vi "Destroy Events.vi"(8 "error in (no error)":errorcluster, 11 "RPI.SenseHat.Actor in":refnum<class "RPI.SenseHat.Actor.lvclass">) -> (0 "error out":errorcluster, 3 "RPI.SenseHat.Actor out":refnum<class "RPI.SenseHat.Actor.lvclass">)   [LabVIEW 2020, in "RPI.SenseHat.Actor.lvlib" / "RPI.SenseHat.Actor.lvclass"]
uses:
  RPI.SenseHat.Actor.lvclass
  RPI.SenseHat.Actor.lvclass/RPI.SenseHat.Actor.ctl
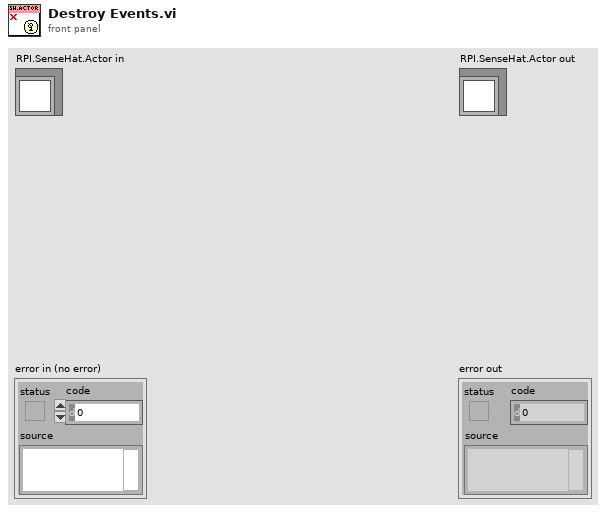
[diagram p1: front panel]
types:
  T1 = typedef "RPI.SenseHat.Actor.lvlib/RPI.SenseHat.Actor.lvclass/Public Events.ctl" = cluster{"Joystick Update":refnum<user-event>}
  T2 = typedef "RPI.SenseHat.Actor.lvlib/RPI.SenseHat.Actor.lvclass/Protected Events.ctl" = cluster{"StopActor":refnum<user-event>}
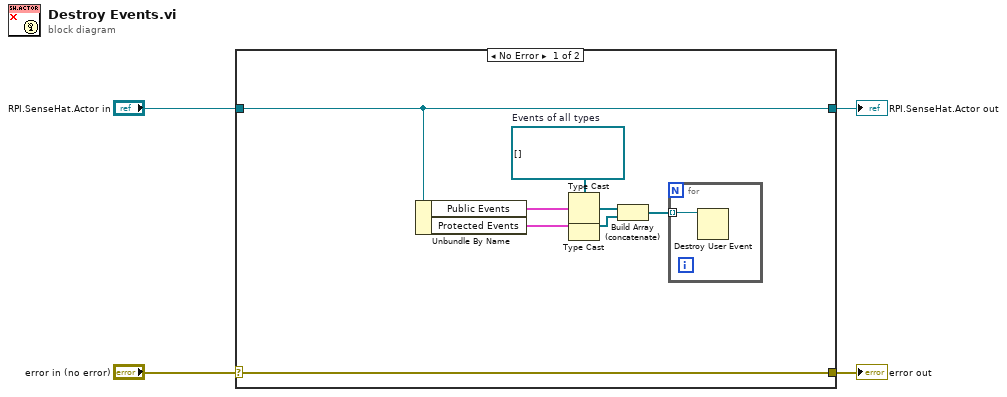
[diagram p0: block diagram]
diagram:
  n1 = case shown="No Error" "error in (no error)" {
    selector: "error in (no error)" -> [w12 w15]
    tunnel: [w12 w15] -> w3
    tunnel: [w11 w14] -> w1
    tunnel: "RPI.SenseHat.Actor in" -> [w11 w14]
    frame No Error {
      w7 = refnum<user-event>[] []  # Events of all types
      n2 = Unbundle By Name(w11) -> ("Public Events"=w10:T1, "Protected Events"=w8:T2)
      n3 = Type Cast(type=w7, x=w10) -> (*(type *) &x=w9:refnum<user-event>[])
      n4 = Type Cast(type=w7, x=w8) -> (*(type *) &x=w5:refnum<user-event>[])
      n5 = Build Array (concatenate)(w9, w5) -> (w6:refnum<user-event>[])
      n6 = for {
        tunnel: w6 -> [w13] mode=indexing
        n7 = Destroy User Event(user event=w13) -> ()  [unwired: 1 in, 1 out]
      }
    }
    frame Error {
    }
  }
  "error out" <- w3
  "RPI.SenseHat.Actor out" <- w1
